vi "Project Parser_Identify External Folders and Internal Relative Paths.vi"(7 "To Lower Case?(T)":bool=TRUE, 8 "error in (no error)":errorcluster, 10 "Project Files":string[](array[string]), 11 "Project Path in":path) -> (0 "error out":errorcluster, 2 "Internal Relative Paths":string[](array[string]), 3 "External Folder Combinations":string[](array[string]))   [LabVIEW 2019, in "Project.Dependencies Finder.lvlib"]
doc: "Split 'Project Files' into array of 'Internal Relative Paths' and 'External Folder Names'.\n\n2020-11-13: Henrik Dueholm Hansen"
uses:
  8584cef7-6435-468f-b24b-0a43cbeddf19.vi
  adfe3204-eb0e-4237-ad1b-a1e7be6d89d0.vi
  Project.Dependencies Finder.lvlib
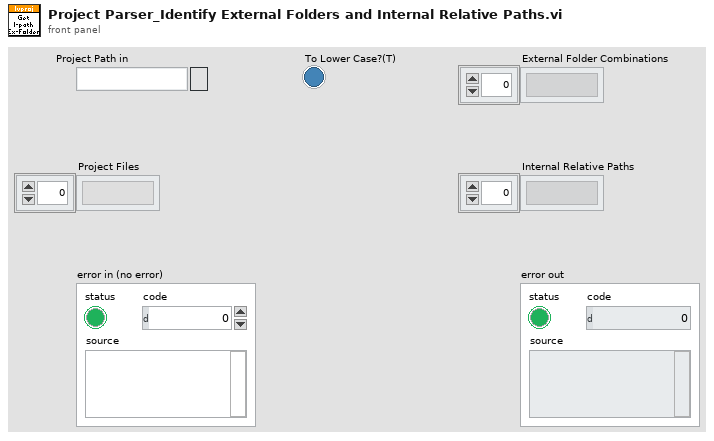
[diagram p1: front panel]
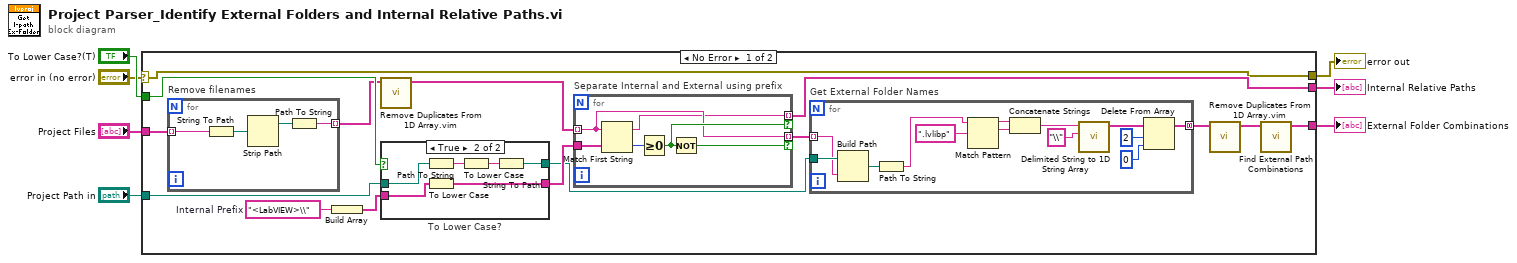
[diagram p0: block diagram]
diagram:
  n1 = case shown="No Error" "error in (no error)" {
    selector: "error in (no error)" -> [w10 w54]
    tunnel: "To Lower Case?(T)" -> [w22 _]
    tunnel: "Project Files" -> [w21 _]
    tunnel: "Project Path in" -> [w20 _]
    tunnel: [w19 _] -> w4
    tunnel: [w8 _] -> w3
    tunnel: [w10 w54] -> w1
    frame No Error {
      w12 = "<LabVIEW>\\"  # Internal Prefix
      n2 = for "Remove filenames" {
        tunnel: w21 -> [w53] mode=indexing
        tunnel: [w50] -> w18 mode=indexing
        n3 = String To Path(string=w53) -> (path=w52:path)
        n4 = Strip Path(path=w52) -> (stripped path=w51:path)  [unwired: 1 out]
        n5 = Path To String(path=w51) -> (string=w50:string)
      }
      n6 = Build Array(w12) -> (w11:string[])
      n7 = call "Remove Duplicates From 1D Array.vim"("array"=w18) -> ("array with duplicates removed"=w17:string[])  [unwired: 10 in]
      n8 = case "To Lower Case?" shown="True" w22 {
        tunnel: [w24 w28] -> w16
        tunnel: [w23 w27] -> w14
        tunnel: w20 -> [w23 w26]
        tunnel: w11 -> [w24 w25]
        frame False {
        }
        frame True {
          n9 = Path To String(path=w26) -> (string=w30:string)
          n10 = To Lower Case(string=w25) -> (all lower case string=w28:string[])
          n11 = To Lower Case(string=w30) -> (all lower case string=w29:string)
          n12 = String To Path(string=w29) -> (path=w27:path)
        }
      }
      n13 = for "Separate Internal and External using prefix" {
        tunnel: w17 -> [w47] mode=indexing
        tunnel: [w44] -> w19 mode=indexing if=w48
        tunnel: [w47] -> w13 mode=indexing if=w46
        tunnel: w16 -> [w45]
        n14 = Match First String(2:w45, 3:w47) -> (0:w49:i32, 1:w44:string)
        n15 = Greater Or Equal To 0?(x=w49) -> (x >= 0?=w48:bool)
        n16 = Not(x=w48) -> (.not. x?=w46:bool)
      }
      n17 = for "Get External Folder Names" {
        tunnel: w14 -> [w42]
        tunnel: w13 -> [w41] mode=indexing
        tunnel: [w36] -> w15 mode=concatenating
        n18 = Build Path(base path=w42, name or relative path=w41) -> (appended path=w43:path)
        n19 = Path To String(path=w43) -> (string=w34:string)
        n20 = Match Pattern(string=w34, regular expression=".lvlibp") -> (before substring=w33:string, match substring=w31:string)  [unwired: 1 in, 2 out]
        n21 = Concatenate Strings(w33, w31) -> (w32:string)
        n22 = call <vilib>:"Delimited String to 1D String Array.vi"("delimiter"="\\" ("search string/char (-)"), "delimited string"=w32) -> ("string array"=w40:string[])  [unwired: 9 in]
        n23 = Delete From Array(array=w40, length=2, index=0) -> (array with subset deleted=w36:string[])  [unwired: 1 out]
      }
      n24 = call "Remove Duplicates From 1D Array.vim"("array"=w15) -> ("array with duplicates removed"=w9:string[])  [unwired: 10 in]
      n25 = call "Find External Path Combinations.vi"("Found Common Paths in"=w9) -> ("External Path Combinations"=w8:string[])  [unwired: 10 in]
    }
    frame Error {
    }
  }
  "error out" <- w1
  "Internal Relative Paths" <- w4
  "External Folder Combinations" <- w3
